vi "Initialize.vi"(6 "Reset (False)":bool, 7 "start path":path, 8 "error in (no error)":errorcluster, 9 "Modbus Address":u16=1 min=1 max=255 step=1, 10 "IP Address":string, 11 "vici_flow_actuator_parent in":refnum<class "heater_parent.lvclass">) -> (0 "error out":errorcluster, 2 "Comms Failure (F: OK)":bool, 3 "vici_flow_actuator_parent out":refnum<class "heater_parent.lvclass">)   [LabVIEW 2020, in "polar_bear_plus_drivers.lvlib" / "heater_parent.lvclass"]
doc: "Establishes communication with the instrument and optionally performs an instrument identification query and/or an instrument reset. It also places the instrument in a default state needed for other instrument driver operations. Therefore, call this VI before calling other instrument driver VIs for this instrument. Generally, you need to call the <b>Initialize</b> VI only once at the beginning of an application."
uses:
  <instrlib>/RxnRover/Driver Polar Bear Plus/heater_parent/heater_parent.lvclass
  <instrlib>/RxnRover/Driver Polar Bear Plus/heater_parent/heater_parent.lvclass/heater_parent.ctl
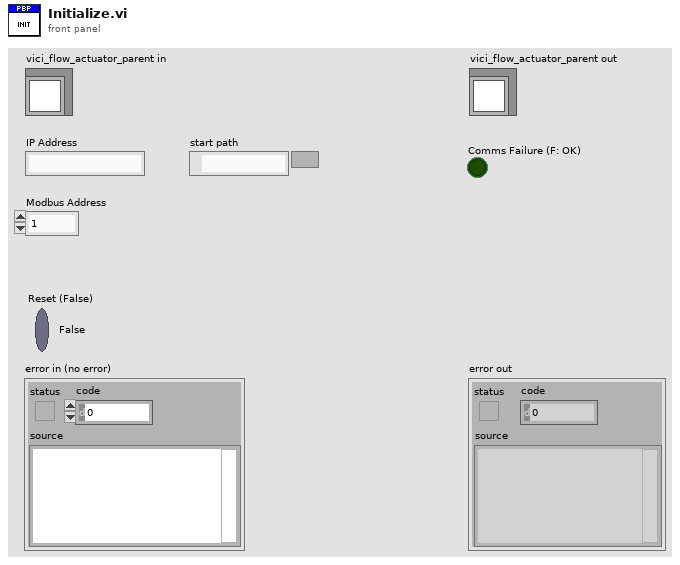
[diagram p1: front panel]
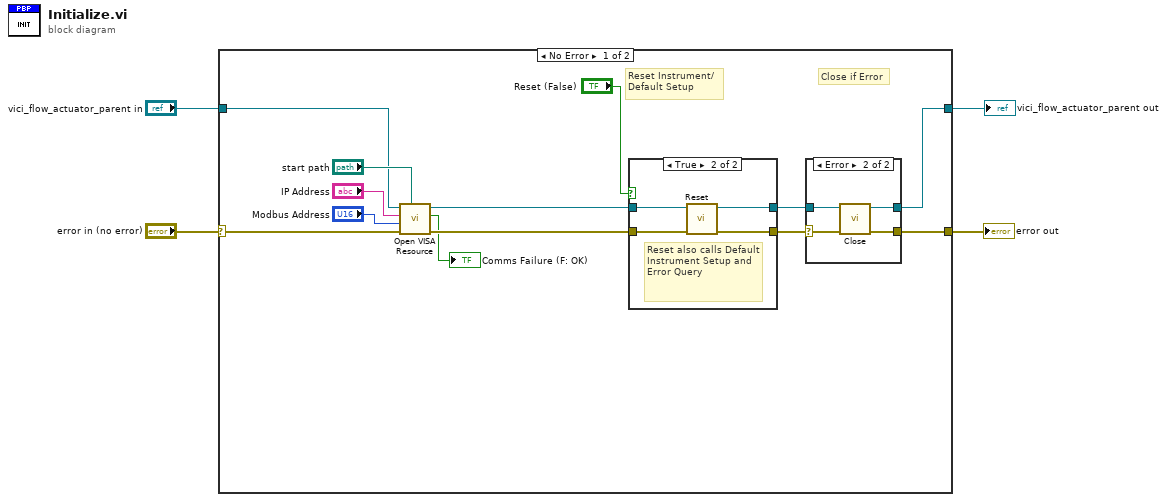
[diagram p0: block diagram]
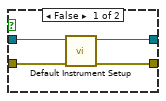
[diagram p3: hidden frame]
diagram:
  n1 = case shown="No Error" "error in (no error)" {
    selector: "error in (no error)" -> [w12 w33]
    tunnel: [w13 w33] -> w3
    tunnel: [w14 w32] -> w1
    tunnel: "vici_flow_actuator_parent in" -> [w7 w32]
    frame No Error {
      # "Close if Error"
      # "Reset Instrument/\nDefault Setup"
      n2 = call-dynamic "Open VISA Resource.vi"("start path"="start path", "error in (no error)"=w12, "Modbus Address"="Modbus Address", "IP Address"="IP Address", "heater_parent in"=w7) -> ("error out"=w11:errorcluster, "Comms Failure"=→"Comms Failure (F: OK)":bool, "heater_parent out"=w6:refnum<class "heater_parent.lvclass">)  [unwired: 4 in]
      n3 = case shown="True" "Reset (False)" {
        tunnel: w11 -> [w26 w29]
        tunnel: [w24 w31] -> w15
        tunnel: w6 -> [w27 w30]
        tunnel: [w25 w28] -> w16
        frame False {
          n4 = call-dynamic "Default Instrument Setup.vi"("error in (no error)"=w26, "heater_parent in"=w27) -> ("error out"=w24:errorcluster, "heater_parent out"=w25:refnum<class "heater_parent.lvclass">)  [unwired: 8 in]
        }
        frame True {
          # "Reset also calls Default Instrument Setup and Error Query"
          n5 = call-dynamic "Reset.vi"("error in (no error)"=w29, "vici_flow_actuator_parent in"=w30) -> ("error out"=w31:errorcluster, "vici_flow_actuator_parent out"=w28:refnum<class "heater_parent.lvclass">)  [unwired: 8 in]
        }
      }
      n6 = case shown="Error" w15 {
        selector: w15 -> [w18 w21]
        tunnel: w16 -> [w19 w22]
        tunnel: [w19 w20] -> w14
        tunnel: [w18 w23] -> w13
        frame No Error {
        }
        frame Error {
          n7 = call-dynamic "Close.vi"("error in (no error)"=w21, "heater_parent in"=w22) -> ("error out"=w23:errorcluster, "heater_parent out"=w20:refnum<class "heater_parent.lvclass">)  [unwired: 8 in]
        }
      }
    }
    frame Error {
    }
  }
  "error out" <- w3
  "vici_flow_actuator_parent out" <- w1
